vi "Agilent E3633 DC PS.vi"   [LabVIEW 2018]
uses:
  <instrlib>/Agilent E363X/Agilent E363X Series.lvlib
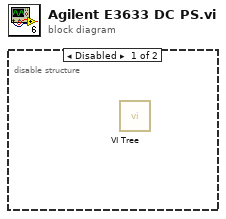
[diagram p0: block diagram]
diagram:
  n1 = disable-structure shown="Disabled" {
    frame Disabled {
      n2 = call <instrlib>:"VI Tree.vi"() -> ()  [unwired: 12 in]
    }
    frame Enabled {
    }
  }
